vi "main.vi"(8 "error in (no error)":errorcluster, 11 "post_installer []":refnum<class "lv-post-installer.lvclass">[](array[class])) -> (0 "error out":errorcluster)   [LabVIEW 2015, in "lv-post-installer-interface.lvlib"]
uses:
  lv-post-installer-interface.lvlib
  private/_controls/tab_control.ctl
  private/_controls/navigation.ctl
  lv-post-installer/public/classes/lv-post-installer/lv-post-installer.lvclass
  private/_controls/hmi_references.ctl
  lv-post-installer/public/advanced/load_class-multiple.vi
  <userlib>/antonio-alexander/lv-bin/lv-bin/public/api/v1/advanced/add_data_path_single.vi
  lv-post-installer/lv-post-installer.lvlib
  <userlib>/antonio-alexander/lv-bin/lv-bin/public/api/v1/v1.lvlib
panel:
  in  "exit":bool
  out "software_current":string caption="Software (Current)"
  in  "software_list":i32[](listbox) caption="Software List"
  in  "navigation":T1=enum."automatic"
  in  "tab_control":T2
  in  "automatic_install":bool
  in  "automatic_uninstall":bool
  in  "manual_download":bool
  in  "manual_uninstall":bool
  in  "manual_install":bool
  in  "backup":bool
  in  "migrate":bool
  in  "re-install":bool
  in  "restore":bool
  in  "add_download_path":bool
  in  "add_post_installer":bool
  in  "add_bin_path":bool
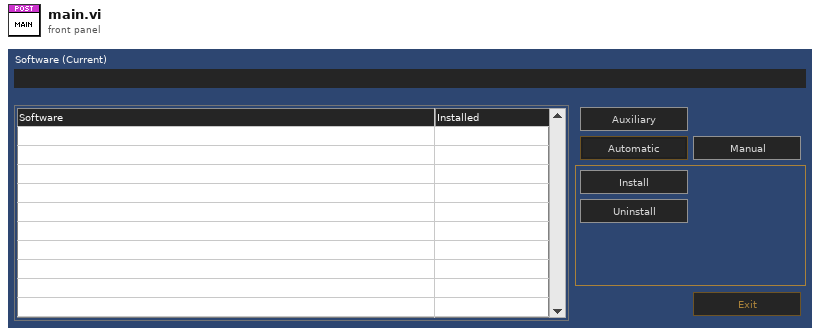
[diagram p1: front panel]
types:
  T1 = typedef "lv-post-installer-interface.lvlib/navigation.ctl" = enum32{"auxiliary", "automatic", "manual"}
  T2 = typedef "lv-post-installer-interface.lvlib/tab_control.ctl" = enum32{"automatic", "manual", "auxiliary"}
  T3 = typedef "lv-post-installer-interface.lvlib/hmi_references.ctl" = cluster{"vi_references":refnum<vi>, "software_list":refnum<vi>, "tab_control":refnum<vi>, "navigation":refnum<vi>, "software_current":refnum<vi>}
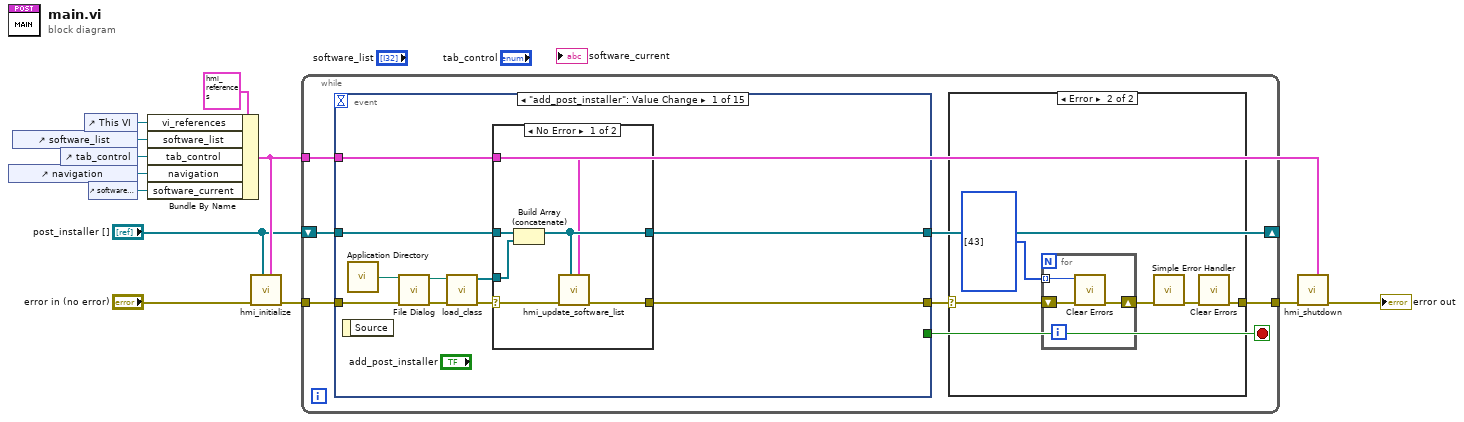
[diagram p0: block diagram]
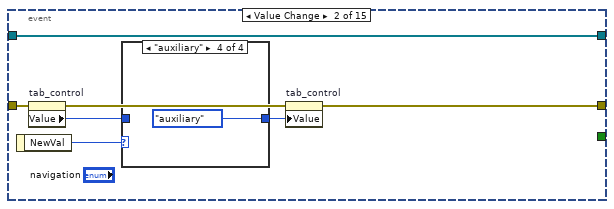
[diagram p3: hidden frame]
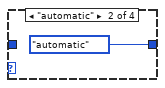
[diagram p5: hidden frame]
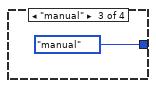
[diagram p6: hidden frame]
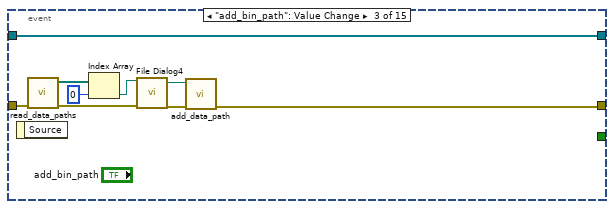
[diagram p7: hidden frame]
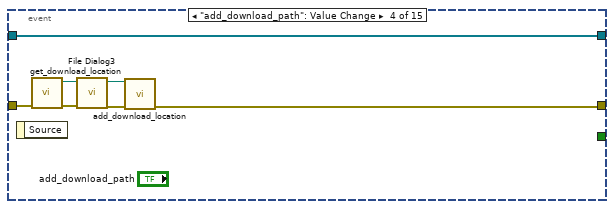
[diagram p8: hidden frame]
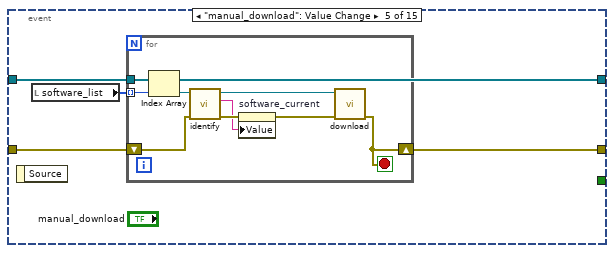
[diagram p9: hidden frame]
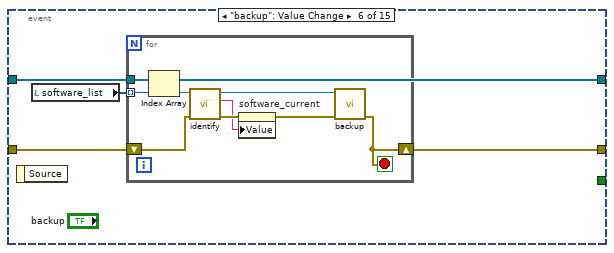
[diagram p10: hidden frame]
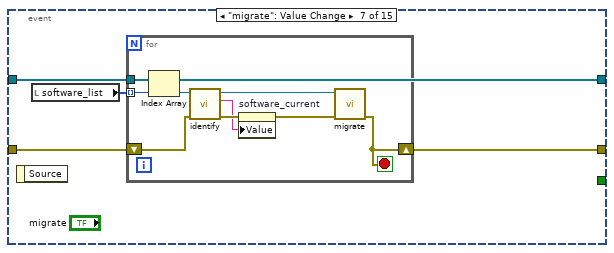
[diagram p11: hidden frame]
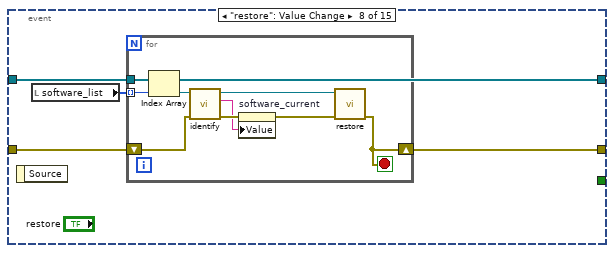
[diagram p12: hidden frame]
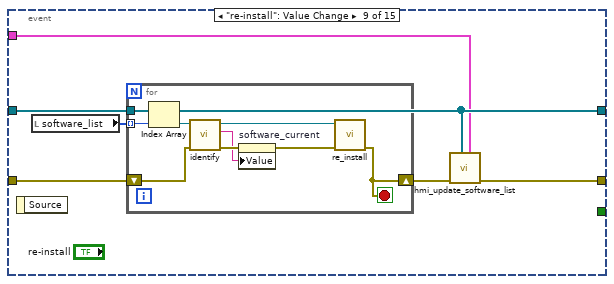
[diagram p13: hidden frame]
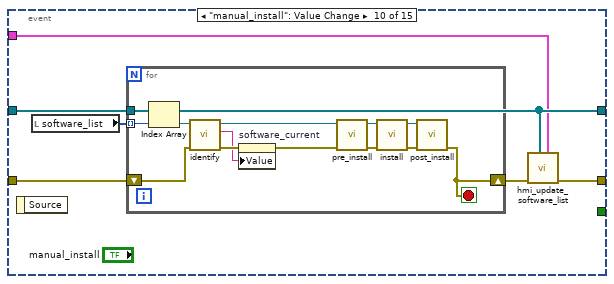
[diagram p14: hidden frame]
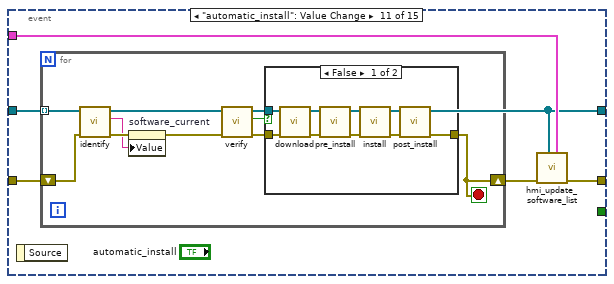
[diagram p15: hidden frame]
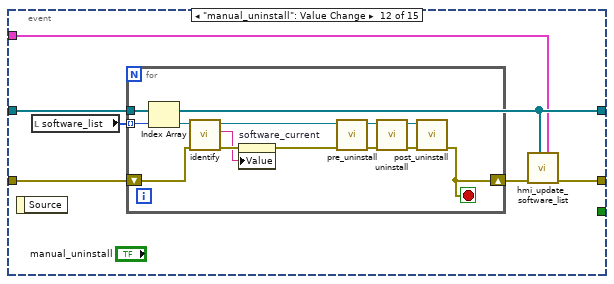
[diagram p17: hidden frame]
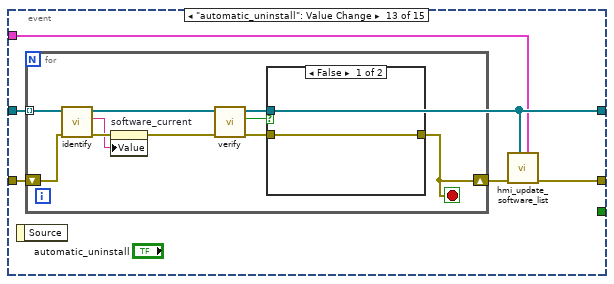
[diagram p18: hidden frame]
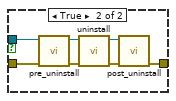
[diagram p19: hidden frame]
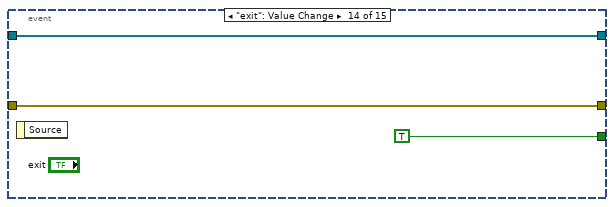
[diagram p20: hidden frame]
diagram:
  n1 = control-ref of="navigation"() -> (w6:refnum<vi>)
  n2 = control-ref of="software_list"() -> (w9:refnum<vi>)
  n3 = control-ref of="tab_control"() -> (w7:refnum<vi>)
  n4 = control-ref of="This VI"() -> (w10:refnum<vi>)
  n5 = control-ref of="software_current"() -> (w2:refnum<vi>)
  n6 = Bundle By Name(cluster=T3 {"vi_references"=refnum, "software_list"=refnum, "tab_control"=refnum, "navigation"=refnum, "software_current"=refnum}, "vi_references"=w10, "software_list"=w9, "tab_control"=w7, "navigation"=w6, "software_current"=w2) -> (w5:T3)
  n7 = call "hmi_initialize.vi"("hmi_references"=w5, "post_installer []"="post_installer []", "error in (no error)"="error in (no error)") -> ("error out"=w12:errorcluster)  [unwired: 8 in]
  n8 = while {
    tunnel: w12 -> [w18]
    tunnel: [w13] -> w3
    shift-right: [w16] -> _
    shift-left: "post_installer []" -> [w17]
    tunnel: w5 -> [w15]
    stop <- w19 stop-if-true
    n9 = event shown="[0] \"add_post_installer\": Value Change" {
      selector: _ -> [_ _ _ _ _ _ _ _ _ _ _ _ _ _ _]
      dyn-events: _ -> [_ _ _ _ _ _ _ _ _ _ _ _ _ _ _]
      timeout: _ -> [_ _ _ _ _ _ _ _ _ _ _ _ _ _ _]
      tunnel: [_ _ _ _ _ _ _ _ _ _ _ _ _ TRUE w221] -> w19
      tunnel: w18 -> [w27 w43 w51 w59 w66 w79 w92 w105 w121 w136 w155 w180 w199 w219 w223]
      tunnel: [w21 w40 w54 w61 w65 w78 w91 w104 w117 w134 w153 w178 w195 w219 w223] -> w14
      tunnel: w17 -> [w26 w44 w57 w64 w67 w80 w93 w106 w120 w133 w151 w177 w198 w218 w222]
      tunnel: [w25 w44 w57 w64 w67 w80 w93 w106 w120 w133 w151 w177 w198 w218 w222] -> w16
      tunnel: w15 -> [w22 _ _ _ _ _ _ _ w119 w132 w152 w176 w197 _ _]
      event "add_post_installer": Value Change {
        n10 = event-data() -> ()  [unwired: 1 in, 1 out]
        n11 = call <vilib>:"Application Directory.vi"() -> ("Application Directory"=w20:path)
        n12 = call "File Dialog"("start path"=w20, "error in"=w27) -> ("selected path"=w28:path, "error out"=w29:errorcluster)  [unwired: 10 in, 2 out]
        n13 = call-poly "load_class.vi"("error in (no error)"=w29, "class_folder"=w28) -> ("error out"=w23:errorcluster, "lv_post_installer []"=w24:refnum<class "lv-post-installer.lvclass">[])  [unwired: 8 in]
        n14 = case shown="No Error" w23 {
          selector: w23 -> [w33 w36]
          tunnel: w26 -> [w35 w37]
          tunnel: [w31 w37] -> w25
          tunnel: w24 -> [w34 _]
          tunnel: [w32 w36] -> w21
          tunnel: w22 -> [w30 _]
          frame No Error {
            n15 = Build Array (concatenate)(w35, w34) -> (w31:refnum<class "lv-post-installer.lvclass">[])
            n16 = call "hmi_update_software_list.vi"("hmi_references"=w30, "post_installer []"=w31, "error in (no error)"=w33) -> ("error out"=w32:errorcluster)  [unwired: 8 in]
          }
          frame Error {
          }
        }
      }
      event Value Change {
        n17 = event-data() -> ("NewVal"=w38:T1)  [unwired: 1 in]
        n18 = property on="tab_control" class="TabCtl (strict)"(error in=w43) -> (error out=w41:errorcluster, "Value"=w42:T2)  [unwired: 1 in, 1 out]
        n19 = case shown="\"auxiliary\"" w38 {
          tunnel: w42 -> [w45 _ _ _]
          tunnel: [w45 tab_control."automatic" ("Value") tab_control."manual" ("Value") tab_control."auxiliary" ("Value")] -> w39
          frame Default {
          }
          frame "automatic" {
          }
          frame "manual" {
          }
          frame "auxiliary" {
          }
        }
        n20 = property on="tab_control" class="TabCtl (strict)"(error in=w41, "Value"=w39) -> (error out=w40:errorcluster)  [unwired: 1 in, 1 out]
      }
      event "add_bin_path": Value Change {
        n21 = event-data() -> ()  [unwired: 1 in, 1 out]
        n22 = call <userlib>:"read_data_paths.vi"("error in (no error)"=w51) -> ("error out"=w50:errorcluster, "path [] out"=w53:path[])  [unwired: 9 in]
        n23 = Index Array(array=w53, index=0) -> (element=w52:path)
        n24 = call "File Dialog4"("start path"=w52, "error in"=w50) -> ("selected path"=w56:path, "error out"=w55:errorcluster)  [unwired: 10 in, 2 out]
        n25 = call-poly <userlib>:"add_data_path.vi"("error in (no error)"=w55, "path_to_add"=w56) -> ("error out"=w54:errorcluster)  [unwired: 9 in]
      }
      event "add_download_path": Value Change {
        n26 = event-data() -> ()  [unwired: 1 in, 1 out]
        n27 = call "get_download_location.vi"("error in (no error)"=w59) -> ("error out"=w58:errorcluster, "download_location"=w60:path)  [unwired: 9 in]
        n28 = call "File Dialog3"("start path"=w60, "error in"=w58) -> ("selected path"=w63:path, "error out"=w62:errorcluster)  [unwired: 10 in, 2 out]
        n29 = call "add_download_location.vi"("error in (no error)"=w62, "path"=w63) -> ("error out"=w61:errorcluster)  [unwired: 9 in]
      }
      event "manual_download": Value Change {
        n30 = event-data() -> ()  [unwired: 1 in, 1 out]
        n31 = local read "software_list"() -> (w68:i32[])
        n32 = for {
          tunnel: w68 -> [w76] mode=indexing
          tunnel: w67 -> [w77]
          shift-right: [w75] -> w65
          shift-left: w66 -> [w72]
          stop <- w75 stop-if-true
          n33 = Index Array(array=w77, index=w76) -> (element=w74:refnum<class "lv-post-installer.lvclass">)
          n34 = call-dynamic "identify.vi"("error in (no error)"=w72, "plugin_interface in"=w74) -> ("error out"=w71:errorcluster, "identifier"=w70:string, "plugin_interface out"=w73:refnum<class "lv-post-installer.lvclass">)  [unwired: 7 in]
          n35 = property on="software_current" class="Str"(error in=w71, "Value"=w70) -> (error out=w69:errorcluster)  [unwired: 1 in, 1 out]
          n36 = call-dynamic "download.vi"("error in (no error)"=w69, "plugin_interface in"=w73) -> ("error out"=w75:errorcluster)  [unwired: 8 in, 1 out]
        }
      }
      event "backup": Value Change {
        n37 = event-data() -> ()  [unwired: 1 in, 1 out]
        n38 = local read "software_list"() -> (w81:i32[])
        n39 = for {
          tunnel: w81 -> [w89] mode=indexing
          tunnel: w80 -> [w90]
          shift-right: [w88] -> w78
          shift-left: w79 -> [w85]
          stop <- w88 stop-if-true
          n40 = Index Array(array=w90, index=w89) -> (element=w87:refnum<class "lv-post-installer.lvclass">)
          n41 = call-dynamic "identify.vi"("error in (no error)"=w85, "plugin_interface in"=w87) -> ("error out"=w84:errorcluster, "identifier"=w83:string, "plugin_interface out"=w86:refnum<class "lv-post-installer.lvclass">)  [unwired: 7 in]
          n42 = property on="software_current" class="Str"(error in=w84, "Value"=w83) -> (error out=w82:errorcluster)  [unwired: 1 in, 1 out]
          n43 = call-dynamic "backup.vi"("error in (no error)"=w82, "plugin_interface in"=w86) -> ("error out"=w88:errorcluster)  [unwired: 8 in, 1 out]
        }
      }
      event "migrate": Value Change {
        n44 = event-data() -> ()  [unwired: 1 in, 1 out]
        n45 = local read "software_list"() -> (w94:i32[])
        n46 = for {
          tunnel: w94 -> [w102] mode=indexing
          tunnel: w93 -> [w103]
          shift-right: [w101] -> w91
          shift-left: w92 -> [w98]
          stop <- w101 stop-if-true
          n47 = Index Array(array=w103, index=w102) -> (element=w100:refnum<class "lv-post-installer.lvclass">)
          n48 = call-dynamic "identify.vi"("error in (no error)"=w98, "plugin_interface in"=w100) -> ("error out"=w97:errorcluster, "identifier"=w96:string, "plugin_interface out"=w99:refnum<class "lv-post-installer.lvclass">)  [unwired: 7 in]
          n49 = property on="software_current" class="Str"(error in=w97, "Value"=w96) -> (error out=w95:errorcluster)  [unwired: 1 in, 1 out]
          n50 = call-dynamic "migrate.vi"("error in (no error)"=w95, "plugin_interface in"=w99) -> ("error out"=w101:errorcluster)  [unwired: 8 in, 1 out]
        }
      }
      event "restore": Value Change {
        n51 = event-data() -> ()  [unwired: 1 in, 1 out]
        n52 = local read "software_list"() -> (w107:i32[])
        n53 = for {
          tunnel: w107 -> [w115] mode=indexing
          tunnel: w106 -> [w116]
          shift-right: [w114] -> w104
          shift-left: w105 -> [w111]
          stop <- w114 stop-if-true
          n54 = Index Array(array=w116, index=w115) -> (element=w113:refnum<class "lv-post-installer.lvclass">)
          n55 = call-dynamic "identify.vi"("error in (no error)"=w111, "plugin_interface in"=w113) -> ("error out"=w110:errorcluster, "identifier"=w109:string, "plugin_interface out"=w112:refnum<class "lv-post-installer.lvclass">)  [unwired: 7 in]
          n56 = property on="software_current" class="Str"(error in=w110, "Value"=w109) -> (error out=w108:errorcluster)  [unwired: 1 in, 1 out]
          n57 = call-dynamic "restore.vi"("error in (no error)"=w108, "plugin in"=w112) -> ("error out"=w114:errorcluster)  [unwired: 8 in, 1 out]
        }
      }
      event "re-install": Value Change {
        n58 = event-data() -> ()  [unwired: 1 in, 1 out]
        n59 = local read "software_list"() -> (w122:i32[])
        n60 = for {
          tunnel: w122 -> [w130] mode=indexing
          tunnel: w120 -> [w131]
          shift-right: [w129] -> w118
          shift-left: w121 -> [w126]
          stop <- w129 stop-if-true
          n61 = Index Array(array=w131, index=w130) -> (element=w128:refnum<class "lv-post-installer.lvclass">)
          n62 = call-dynamic "identify.vi"("error in (no error)"=w126, "plugin_interface in"=w128) -> ("error out"=w125:errorcluster, "identifier"=w124:string, "plugin_interface out"=w127:refnum<class "lv-post-installer.lvclass">)  [unwired: 7 in]
          n63 = property on="software_current" class="Str"(error in=w125, "Value"=w124) -> (error out=w123:errorcluster)  [unwired: 1 in, 1 out]
          n64 = call-dynamic "re_install.vi"("error in (no error)"=w123, "post_installer-interface in"=w127) -> ("error out"=w129:errorcluster)  [unwired: 8 in, 1 out]
        }
        n65 = call "hmi_update_software_list.vi"("hmi_references"=w119, "post_installer []"=w120, "error in (no error)"=w118) -> ("error out"=w117:errorcluster)  [unwired: 8 in]
      }
      event "manual_install": Value Change {
        n66 = event-data() -> ()  [unwired: 1 in, 1 out]
        n67 = local read "software_list"() -> (w137:i32[])
        n68 = for {
          tunnel: w137 -> [w149] mode=indexing
          tunnel: w133 -> [w150]
          shift-right: [w141] -> w135
          shift-left: w136 -> [w147]
          stop <- w141 stop-if-true
          n69 = Index Array(array=w150, index=w149) -> (element=w148:refnum<class "lv-post-installer.lvclass">)
          n70 = call-dynamic "identify.vi"("error in (no error)"=w147, "plugin_interface in"=w148) -> ("error out"=w146:errorcluster, "identifier"=w145:string, "plugin_interface out"=w144:refnum<class "lv-post-installer.lvclass">)  [unwired: 7 in]
          n71 = property on="software_current" class="Str"(error in=w146, "Value"=w145) -> (error out=w138:errorcluster)  [unwired: 1 in, 1 out]
          n72 = call-dynamic "pre_install.vi"("error in (no error)"=w138, "plugin_interface in"=w144) -> ("error out"=w139:errorcluster, "plugin_interface out"=w140:refnum<class "lv-post-installer.lvclass">)  [unwired: 8 in]
          n73 = call-dynamic "install.vi"("error in (no error)"=w139, "plugin_interface in"=w140) -> ("error out"=w143:errorcluster, "plugin_interface out"=w142:refnum<class "lv-post-installer.lvclass">)  [unwired: 8 in]
          n74 = call-dynamic "post_install.vi"("error in (no error)"=w143, "plugin_interface in"=w142) -> ("error out"=w141:errorcluster)  [unwired: 8 in, 1 out]
        }
        n75 = call "hmi_update_software_list.vi"("hmi_references"=w132, "post_installer []"=w133, "error in (no error)"=w135) -> ("error out"=w134:errorcluster)  [unwired: 8 in]
      }
      event "automatic_install": Value Change {
        n76 = event-data() -> ()  [unwired: 1 in, 1 out]
        n77 = for {
          tunnel: w151 -> [w161] mode=indexing
          shift-right: [w162] -> w154
          shift-left: w155 -> [w165]
          stop <- w162 stop-if-true
          n78 = call-dynamic "identify.vi"("error in (no error)"=w165, "plugin_interface in"=w161) -> ("error out"=w164:errorcluster, "identifier"=w163:string, "plugin_interface out"=w160:refnum<class "lv-post-installer.lvclass">)  [unwired: 7 in]
          n79 = property on="software_current" class="Str"(error in=w164, "Value"=w163) -> (error out=w158:errorcluster)  [unwired: 1 in, 1 out]
          n80 = call-dynamic "verify.vi"("error in (no error)"=w158, "plugin_interface in"=w160) -> ("error out"=w157:errorcluster, "installed?"=w156:bool, "plugin_interface out"=w159:refnum<class "lv-post-installer.lvclass">)  [unwired: 7 in]
          n81 = case shown="False" w156 {
            tunnel: [w172 w175] -> w162
            tunnel: w159 -> [w169 _]
            tunnel: w157 -> [w166 w175]
            frame False {
              n82 = call-dynamic "download.vi"("error in (no error)"=w166, "plugin_interface in"=w169) -> ("error out"=w167:errorcluster, "plugin_interface out"=w168:refnum<class "lv-post-installer.lvclass">)  [unwired: 8 in]
              n83 = call-dynamic "pre_install.vi"("error in (no error)"=w167, "plugin_interface in"=w168) -> ("error out"=w170:errorcluster, "plugin_interface out"=w171:refnum<class "lv-post-installer.lvclass">)  [unwired: 8 in]
              n84 = call-dynamic "install.vi"("error in (no error)"=w170, "plugin_interface in"=w171) -> ("error out"=w174:errorcluster, "plugin_interface out"=w173:refnum<class "lv-post-installer.lvclass">)  [unwired: 8 in]
              n85 = call-dynamic "post_install.vi"("error in (no error)"=w174, "plugin_interface in"=w173) -> ("error out"=w172:errorcluster)  [unwired: 8 in, 1 out]
            }
            frame True {
            }
          }
        }
        n86 = call "hmi_update_software_list.vi"("hmi_references"=w152, "post_installer []"=w151, "error in (no error)"=w154) -> ("error out"=w153:errorcluster)  [unwired: 8 in]
      }
      event "manual_uninstall": Value Change {
        n87 = event-data() -> ()  [unwired: 1 in, 1 out]
        n88 = local read "software_list"() -> (w181:i32[])
        n89 = for {
          tunnel: w181 -> [w193] mode=indexing
          tunnel: w177 -> [w194]
          shift-right: [w182] -> w179
          shift-left: w180 -> [w191]
          stop <- w182 stop-if-true
          n90 = Index Array(array=w194, index=w193) -> (element=w192:refnum<class "lv-post-installer.lvclass">)
          n91 = call-dynamic "identify.vi"("error in (no error)"=w191, "plugin_interface in"=w192) -> ("error out"=w190:errorcluster, "identifier"=w189:string, "plugin_interface out"=w187:refnum<class "lv-post-installer.lvclass">)  [unwired: 7 in]
          n92 = property on="software_current" class="Str"(error in=w190, "Value"=w189) -> (error out=w188:errorcluster)  [unwired: 1 in, 1 out]
          n93 = call-dynamic "pre_uninstall.vi"("error in (no error)"=w188, "plugin_interface in"=w187) -> ("error out"=w186:errorcluster, "plugin_interface out"=w185:refnum<class "lv-post-installer.lvclass">)  [unwired: 8 in]
          n94 = call-dynamic "uninstall.vi"("error in (no error)"=w186, "plugin_interface in"=w185) -> ("error out"=w183:errorcluster, "plugin_interface out"=w184:refnum<class "lv-post-installer.lvclass">)  [unwired: 8 in]
          n95 = call-dynamic "post_uninstall.vi"("error in (no error)"=w183, "plugin_interface in"=w184) -> ("error out"=w182:errorcluster)  [unwired: 8 in, 1 out]
        }
        n96 = call "hmi_update_software_list.vi"("hmi_references"=w176, "post_installer []"=w177, "error in (no error)"=w179) -> ("error out"=w178:errorcluster)  [unwired: 8 in]
      }
      event "automatic_uninstall": Value Change {
        n97 = event-data() -> ()  [unwired: 1 in, 1 out]
        n98 = for {
          tunnel: w198 -> [w205] mode=indexing
          shift-right: [w206] -> w196
          shift-left: w199 -> [w209]
          stop <- w206 stop-if-true
          n99 = call-dynamic "identify.vi"("error in (no error)"=w209, "plugin_interface in"=w205) -> ("error out"=w208:errorcluster, "identifier"=w207:string, "plugin_interface out"=w204:refnum<class "lv-post-installer.lvclass">)  [unwired: 7 in]
          n100 = property on="software_current" class="Str"(error in=w208, "Value"=w207) -> (error out=w203:errorcluster)  [unwired: 1 in, 1 out]
          n101 = call-dynamic "verify.vi"("error in (no error)"=w203, "plugin_interface in"=w204) -> ("error out"=w201:errorcluster, "installed?"=w200:bool, "plugin_interface out"=w202:refnum<class "lv-post-installer.lvclass">)  [unwired: 7 in]
          n102 = case shown="False" w200 {
            tunnel: [w210 w213] -> w206
            tunnel: w202 -> [_ w212]
            tunnel: w201 -> [w210 w211]
            frame False {
            }
            frame True {
              n103 = call-dynamic "pre_uninstall.vi"("error in (no error)"=w211, "plugin_interface in"=w212) -> ("error out"=w217:errorcluster, "plugin_interface out"=w216:refnum<class "lv-post-installer.lvclass">)  [unwired: 8 in]
              n104 = call-dynamic "uninstall.vi"("error in (no error)"=w217, "plugin_interface in"=w216) -> ("error out"=w214:errorcluster, "plugin_interface out"=w215:refnum<class "lv-post-installer.lvclass">)  [unwired: 8 in]
              n105 = call-dynamic "post_uninstall.vi"("error in (no error)"=w214, "plugin_interface in"=w215) -> ("error out"=w213:errorcluster)  [unwired: 8 in, 1 out]
            }
          }
        }
        n106 = call "hmi_update_software_list.vi"("hmi_references"=w197, "post_installer []"=w198, "error in (no error)"=w196) -> ("error out"=w195:errorcluster)  [unwired: 8 in]
      }
      event "exit": Value Change {
        n107 = event-data() -> ()  [unwired: 1 in, 1 out]
      }
      event Panel Close? {
        w221 = TRUE
        n108 = event-data() -> ()  [unwired: 1 in, 1 out]
        n109 = event-data("Discard?"=w221) -> ()  [unwired: 1 in, 1 out]
      }
    }
    n110 = case shown="Error" w14 {
      selector: w14 -> [w224 w229]
      tunnel: [w224 w225] -> w13
      frame No Error {
      }
      frame Error {
        n111 = for {
          shift-right: [w231] -> w226
          shift-left: w229 -> [w232]
          tunnel: i32[] [43] ("specific error code to clear (0: all)") -> [w230] mode=indexing
          n112 = call <vilib>:"Clear Errors.vi"("error in (no error)"=w232, "specific error code to clear (0: all)"=w230) -> ("error out"=w231:errorcluster)  [unwired: 4 in, 1 out]
        }
        n113 = call <vilib>:"Simple Error Handler.vi"("error in (no error)"=w226) -> ("error out"=w227:errorcluster)  [unwired: 4 in, 4 out]
        n114 = call <vilib>:"Clear Errors.vi"("error in (no error)"=w227) -> ("error out"=w225:errorcluster)  [unwired: 5 in, 1 out]
      }
    }
  }
  n115 = call "hmi_shutdown.vi"("hmi_references"=w5, "error in (no error)"=w3) -> ("error out"=→"error out":errorcluster)  [unwired: 9 in]
